vi "Initialize-lasing-control.vi"(8 "error in (no error)":errorcluster, 11 "TP-Data in":T1) -> (0 "error out":errorcluster, 3 "TP-Data out":T1)   [LabVIEW 2013, in "SLMControl.lvlib" / "SC-Main.lvclass"]
uses:
  SC-Main.lvclass
  Object-reference.ctl
  SM1000/TCP-settings.ctl
  SM1000/DOTNET-settings.ctl
  SM1000/Device-identification.ctl
  SC-Main.lvclass/SC-Main.ctl
  SM1000/SM1000.lvclass
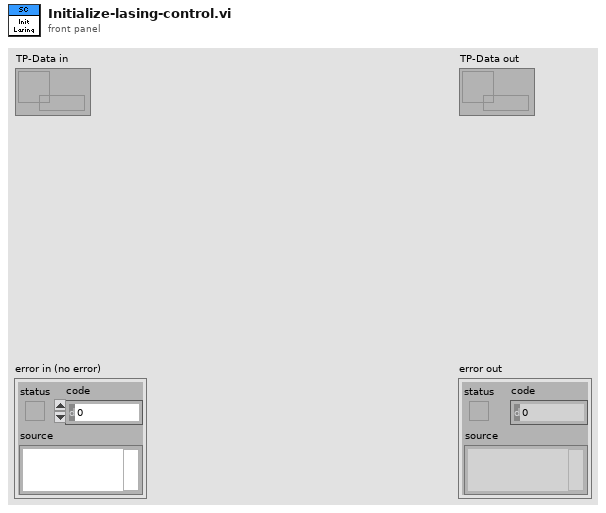
[diagram p1: front panel]
types:
  T1 = typedef "SLMControl.lvlib/SC-Main.lvclass/Object-reference.ctl" = refnum<data-value>
  T2 = typedef "SLMControl.lvlib/SM1000.lvclass/DOTNET-settings.ctl" = cluster{"Target IP":string, "Target broadcast port":i32, "Target communication port":i32, "clientID":i32, "Broadcast IP":string, "Servercount":i32, "Device IDs":T3[]}
  T3 = typedef "SLMControl.lvlib/SM1000.lvclass/Device-identification.ctl" = cluster{"Name":string, "IP":string, "Mac address":string}
  T4 = typedef "SLMControl.lvlib/SM1000.lvclass/TCP-settings.ctl" = cluster{"Target IP":string, "Target TCP port":u16, "TCP read mode":enum16{"Standard", "Buffered", "CRLF", "Immediate"}, "TCP read buffer":i32, "Read timeout":i32}
  T5 = typedef "SLMControl.lvlib/SM1000.lvclass/Object-reference.ctl" = refnum<data-value>
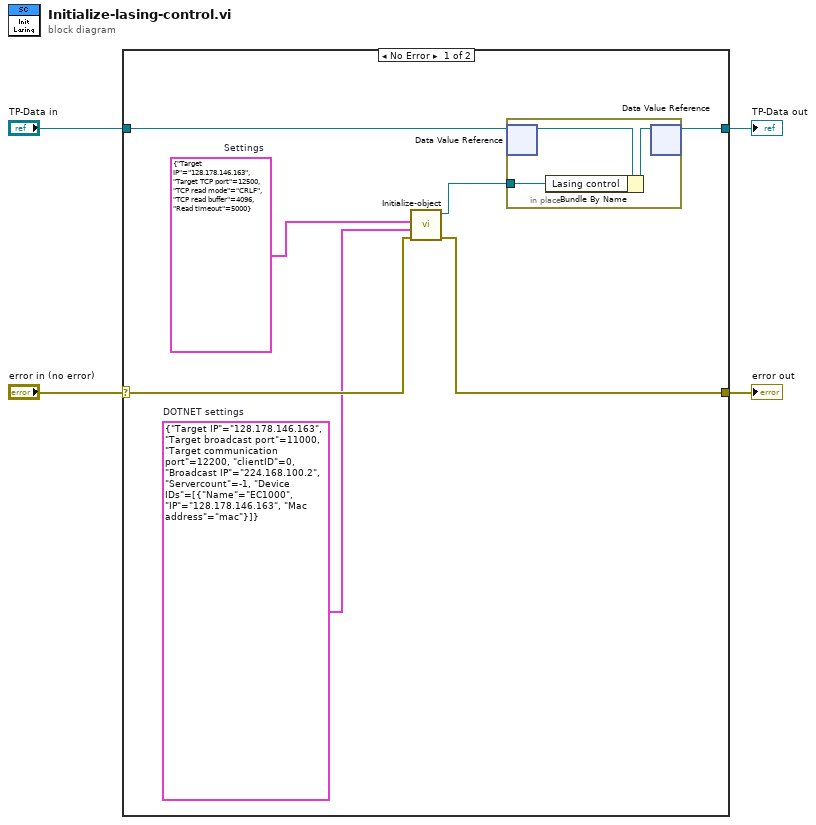
[diagram p0: block diagram]
diagram:
  n1 = case shown="No Error" "error in (no error)" {
    selector: "error in (no error)" -> [w7 w16]
    tunnel: [w8 w16] -> w3
    tunnel: [w10 w15] -> w1
    tunnel: "TP-Data in" -> [w11 w15]
    frame No Error {
      w5 = T2 {"Target IP"="128.178.146.163", "Target broadcast port"=11000, "Target communication port"=12200, "clientID"=0, "Broadcast IP"="224.168.100.2", "Servercount"=-1, "Device IDs"=[{"Name"="EC1000", "IP"="128.178.146.163", "Mac address"="mac"}]}  # DOTNET settings
      w6 = T4 {"Target IP"="128.178.146.163", "Target TCP port"=12500, "TCP read mode"=enum."CRLF", "TCP read buffer"=4096, "Read timeout"=5000}  # Settings
      n2 = call "Initialize-object.vi"("error in (no error)"=w7, "DOTNET settings"=w5, "TCP settings"=w6) -> ("error out"=w8:errorcluster, "SM1000-control out"=w9:T5)  [unwired: 7 in]
      n3 = in-place {
        in-place-border: w9 -> [w12]
        n4 = in-place-dvr #1(w11) -> (w14:refnum<class "SC-Main.lvclass">)  [unwired: 1 out]
        n5 = Bundle By Name(cluster=w14, "Lasing control"=w12) -> (w13:refnum<class "SC-Main.lvclass">)
        n6 = in-place-dvr #1(w13) -> (w10:T1)  [unwired: 1 out]
      }
    }
    frame Error {
    }
  }
  "error out" <- w3
  "TP-Data out" <- w1
